vi "AnalyzerSettings.vi"(8 "ErrorIn":errorcluster, 9 "Set default thresholds? [F]":bool) -> (0 "ErrorOut":errorcluster={"status"=TRUE, "code"=1073, "source"="Invoke Node in SetThresholds.vi->master.vi->main.vi\n<APPEND>\nMethod Name: <b>Default Values:Make Current Default</b>"})   [LabVIEW 2019]
uses:
  MobileAnalyzer/mainVIs/utilities/FGVAction.ctl
  MobileAnalyzer/mainVIs/analyzeAccelerationDataVIs/calculateFaultIndicatorsVIs/Thresholds.ctl
  MobileAnalyzer/mainVIs/analyzeAccelerationDataVIs/calculateFaultIndicatorsVIs/FaultParameter.ctl
  AnalysisSettings.ctl
panel:
  in  "Kurtoza":dbl=5.0 min=0.0
  in  "RMS":dbl=0.3 min=0.0
  in  "Czêstotliwoœci [Hz] i progi":dbl[][](array[numeric])=[[50.0, 0.5]] min=0.0
  in  "Zapisaæ wyniki analizy w analizatorze?":bool=TRUE
  in  "Nazwa serii pomiarowej:":string="Analiza"
  in  "Close":bool
  # "Ustaw wartoœci progów parametrów:"
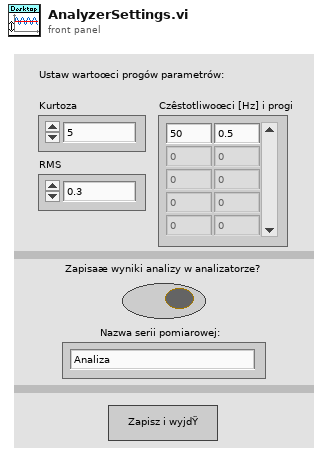
[diagram p1: front panel]
types:
  T1 = typedef "FGVAction.ctl" = enum16{"Read", "Write"}
  T2 = typedef "AnalysisSettings.ctl" = cluster{"Fault Thresholds":T3, "Analysis series name":string, "Save data analysis?":bool}
  T3 = typedef "Thresholds.ctl" = cluster{"Parameters labels":T4[], "Parameters thresholds":dbl[], "Freqs and thresholds":dbl[][]}
  T4 = typedef "FaultParameter.ctl" = enum16{"Kurtosis", "RMS"}
  T5 = typedef "DesktopAppSettings.ctl" = cluster{"MobileAnalyzer IP":string, "Network Stream Timeout Code":i32, "Endpoint Destroyed Code":i32, "Save to file?":bool, "All threads":T6[], "Connected":bool, "AnalysisSettings":T2}
  T6 = typedef "Thread.ctl" = enum16{"GUI", "communicateWithAnalyzer", "saveDataToTDMS"}
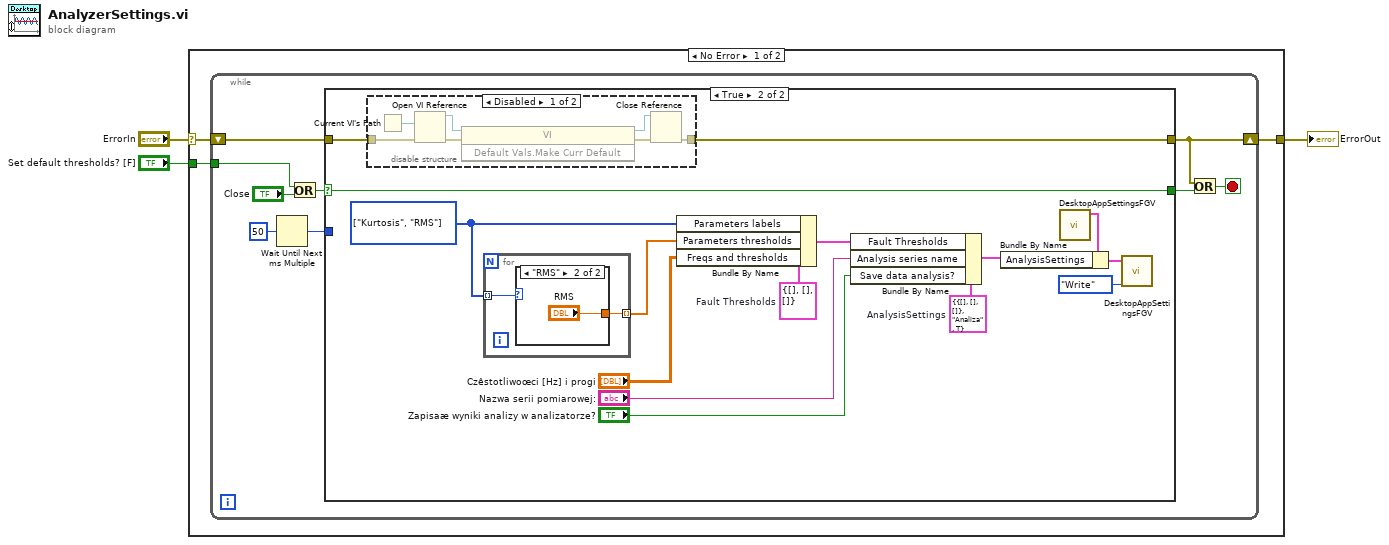
[diagram p0: block diagram]
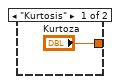
[diagram p3: hidden frame]
diagram:
  n1 = case shown="No Error" "ErrorIn" {
    selector: "ErrorIn" -> [w6 w44]
    tunnel: [w5 w44] -> w2
    tunnel: "Set default thresholds? [F]" -> [w4 _]
    frame No Error {
      n2 = while {
        shift-right: [w9] -> w5
        shift-left: w6 -> [w10]
        tunnel: w4 -> [w7]
        stop <- w15 stop-if-true
        n3 = Wait Until Next ms Multiple(millisecond multiple=u32 50) -> (millisecond timer value=w12:u32)
        n4 = Or(x=w7, y="Close") -> (x .or. y?=w8:bool)
        n5 = case shown="True" w8 {
          selector: w8 -> [_ w31]
          tunnel: w12 -> [_ _]
          tunnel: [_ w31] -> w11
          tunnel: w10 -> [w16 w27]
          tunnel: [w16 w26] -> w9
          frame False {
          }
          frame True {
            w21 = T2 {"Fault Thresholds"={"Parameters labels"=[], "Parameters thresholds"=[], "Freqs and thresholds"=[]}, "Analysis series name"="Analiza", "Save data analysis?"=TRUE}  # AnalysisSettings
            w24 = T4[] [enum."Kurtosis", enum."RMS"] items=["Kurtosis", "RMS"]
            w25 = T3 {"Parameters labels"=[], "Parameters thresholds"=[], "Freqs and thresholds"=[]}  # Fault Thresholds
            n6 = disable-structure shown="Disabled" {
              disable-tunnel: w27 -> [w37 w43]
              disable-tunnel: [w36 w43] -> w26
              frame Disabled {
                n7 = Current VI's Path() -> (path=w38:path)
                n8 = Open VI Reference(vi path=w38, error in (no error)=w37) -> (vi reference=w40:refnum<vi>, error out=w39:errorcluster)  [unwired: 4 in]
                n9 = invoke class="VI" method="Default Vals.Make Curr Default"(reference=w40, error in=w39) -> (reference out=w42:refnum<vi>, error out=w41:errorcluster)  [unwired: 1 in, 1 out]
                n10 = Close Reference(reference=w42, error in (no error)=w41) -> (error out=w36:errorcluster)
              }
              frame Enabled {
              }
            }
            n11 = for {
              tunnel: w24 -> [w33] mode=indexing
              tunnel: [w32] -> w23 mode=indexing
              n12 = case shown="\"RMS\"" w33 {
                tunnel: ["Kurtoza" "RMS"] -> w32
                frame "Kurtosis" {
                }
                frame "RMS" {
                }
              }
            }
            n13 = Bundle By Name(cluster=w25, "Parameters labels"=w24, "Parameters thresholds"=w23, "Freqs and thresholds"="Czêstotliwoœci [Hz] i progi") -> (w20:T3)
            n14 = Bundle By Name(cluster=w21, "Fault Thresholds"=w20, "Analysis series name"="Nazwa serii pomiarowej:", "Save data analysis?"="Zapisaæ wyniki analizy w analizatorze?") -> (w17:T2)
            n15 = call "DesktopAppSettingsFGV.vi"() -> ("DesktopAppSettingsOut"=w29:T5)  [unwired: 11 in]
            n16 = Bundle By Name(cluster=w29, "AnalysisSettings"=w17) -> (w28:T5)
            n17 = call "DesktopAppSettingsFGV.vi"("FGVAction (Read)"=FGVAction."Write", "DesktopAppSettingsIn"=w28) -> ()  [unwired: 9 in, 1 out]
          }
        }
        n18 = Or(x=w9, y=w11) -> (x .or. y?=w15:bool)
      }
    }
    frame Error {
    }
  }
  "ErrorOut" <- w2
